vi "time_waves_graphs.vi"() -> ()   [LabVIEW 2020]
panel:
  out "XY Graph":cluster{dbl[], dbl[]}(graph)
  out "Waveform Graph 2":dynamicdata(graph)
  out "Waveform Graph":cluster{i32, dbl, dbl[]}[](graph)
  in  "stop":bool
  out "Waveform Chart":T1(graph)
  # "Multi Chart of Random Number"
  # "Sphere"
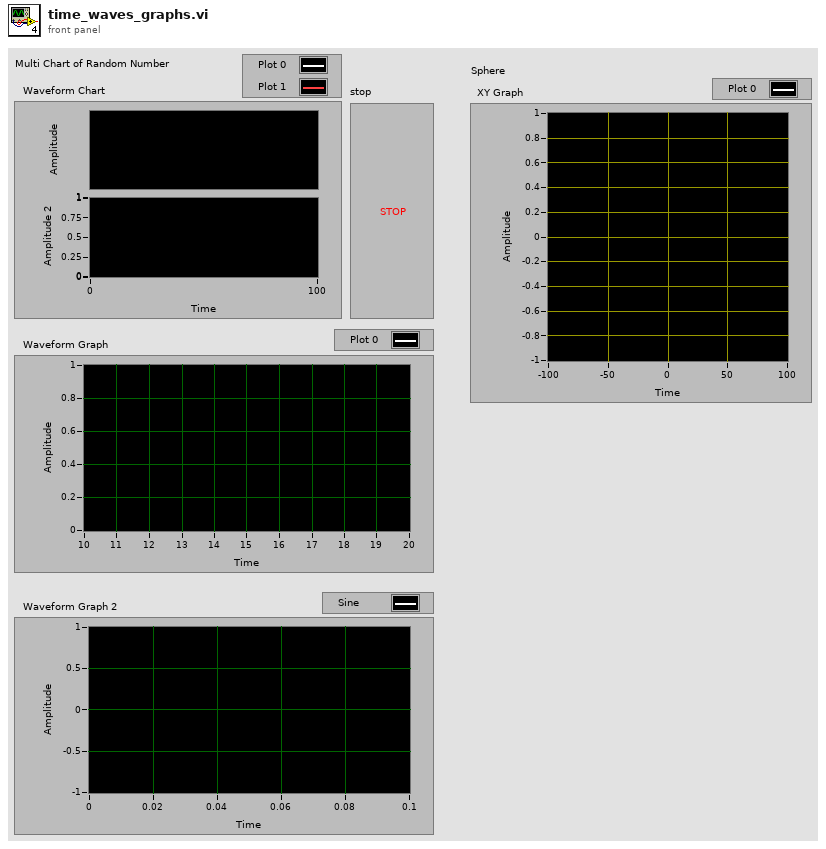
[diagram p1: front panel]
types:
  T1 = cluster{"number: 0 to 1":dbl, "number: 0 to 1":dbl}
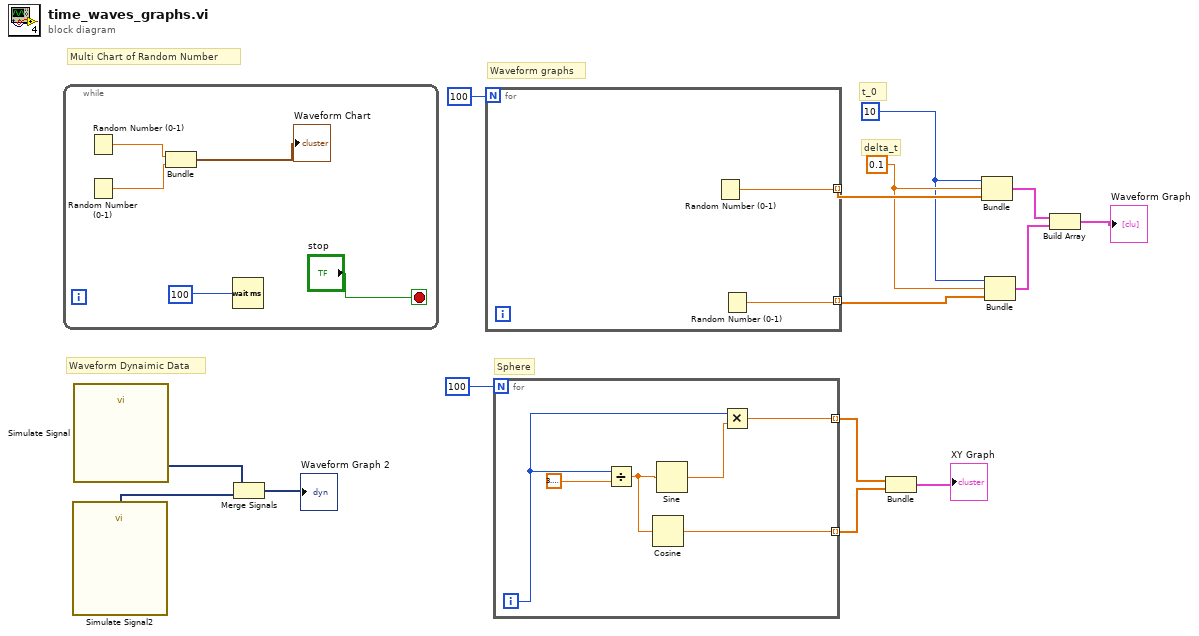
[diagram p0: block diagram]
diagram:
  w11 = 10
  w12 = 0.1
  # "Sphere"
  # "Waveform Dynaimic Data"
  # "t_0"
  # "delta_t"
  # "Waveform graphs"
  # "Multi Chart of Random Number"
  n1 = while {
    stop <- "stop" stop-if-true
    n2 = Random Number (0-1)() -> (number: 0 to 1=w19:dbl)
    n3 = Random Number (0-1)() -> (number: 0 to 1=w18:dbl)
    n4 = Bundle("number: 0 to 1"=w19, "number: 0 to 1"=w18) -> (→"Waveform Chart":T1)  [unwired: 1 in]
    n5 = Wait (ms)(milliseconds to wait=100) -> ()  [unwired: 1 out]
  }
  n6 = call "Simulate Signal2"() -> ("Triangle"=w7:dynamicdata)  [unwired: 14 in, 1 out]
  n7 = call "Simulate Signal"() -> ("Sine"=w6:dynamicdata)  [unwired: 14 in, 1 out]
  n8 = Merge Signals(w6, w7) -> (→"Waveform Graph 2":dynamicdata)
  n9 = for {
    N: 100 -> [_]
    tunnel: [w22] -> w14 mode=indexing
    tunnel: [w21] -> w13 mode=indexing
    n10 = Random Number (0-1)() -> (number: 0 to 1=w21:dbl)
    n11 = Random Number (0-1)() -> (number: 0 to 1=w22:dbl)
  }
  n12 = for {
    N: 100 -> [_]
    tunnel: [w24] -> w3 mode=indexing
    tunnel: [w23] -> w2 mode=indexing
    i -> [w28]
    n13 = Divide(x=w28, y=3.141592653589793) -> (x/y=w26:dbl)
    n14 = Cosine(x=w26) -> (cos(x)=w23:dbl)
    n15 = Sine(x=w26) -> (sin(x)=w25:dbl)
    n16 = Multiply(x=w28, y=w25) -> (x*y=w24:dbl)
  }
  n17 = Bundle(w3, w2) -> (→"XY Graph":cluster{dbl[], dbl[]})  [unwired: 1 in]
  n18 = Bundle(w11, w12, w13) -> (w10:cluster{i32, dbl, dbl[]})  [unwired: 1 in]
  n19 = Bundle(w11, w12, w14) -> (w9:cluster{i32, dbl, dbl[]})  [unwired: 1 in]
  n20 = Build Array(w10, w9) -> (→"Waveform Graph":cluster{i32, dbl, dbl[]}[])
